vi "Agilent Tester.vi"() -> ()   [LabVIEW 2016]
uses:
  Type Definitions/WILT Agilent Data Cluster.ctl
  Type Definitions/WILT Agilent Channel Definition.ctl
panel:
  out "Agilent":T1
  in  "Open/Close (F:Close)":bool=TRUE
  in  "Open Valve":bool
  in  "Station":i32=1
  in  "Agilent Channels In":T2[](array[typedef])=[{"Channel"="301", "Station"="1", "Label"="Water Valve", "Agilent Station"="2", "Data"=0.0}, {"Channel"="302", "Station"="2", "Label"="Water Valve", "Agilent Station"="2", "Data"=0.0}, {"Channel"="303", "Station"="3", "Label"="Water Valve", "Agilent Station"="2", "Data"=0.0}, {"Channel"="304", "Station"="4", "Label"="Water Valve", "Agilent Station"="2", "Data"=0.0}, {"Channel"="305", "Station"="5", "Label"="Water Valve", "Agilent Station"="2", "Data"=0.0}, {"Channel"="306", "Station"="6", "Label"="Water Valve", "Agilent Station"="2", "Data"=0.0}, {"Channel"="307", "Station"="7", "Label"="Water Valve", "Agilent Station"="2", "Data"=0.0}, {"Channel"="308", "Station"="8", "Label"="Water Valve", "Agilent Station"="2", "Data"=0.0}, {"Channel"="309", "Station"="9", "Label"="Water Valve", "Agilent Station"="2", "Data"=0.0}, {"Channel"="310", "Station"="10", "Label"="Water Valve", "Agilent Station"="2", "Data"=0.0}, {"Channel"="311", "Station"="11", "Label"="Water Valve", "Agilent Station"="2", "Data"=0.0}, {"Channel"="312", "Station"="12", "Label"="Water Valve", "Agilent Station"="2", "Data"=0.0}, {"Channel"="313", "Station"="13", "Label"="Water Valve", "Agilent Station"="2", "Data"=0.0}, {"Channel"="314", "Station"="14", "Label"="Water Valve", "Agilent Station"="2", "Data"=0.0}, {"Channel"="315", "Station"="15", "Label"="Water Valve", "Agilent Station"="2", "Data"=0.0}, {"Channel"="316", "Station"="16", "Label"="Water Valve", "Agilent Station"="2", "Data"=0.0}, {"Channel"="317", "Station"="17", "Label"="Water Valve", "Agilent Station"="2", "Data"=0.0}, {"Channel"="318", "Station"="18", "Label"="Water Valve", "Agilent Station"="2", "Data"=0.0}, {"Channel"="319", "Station"="19", "Label"="Water Valve", "Agilent Station"="2", "Data"=0.0}, {"Channel"="320", "Station"="20", "Label"="Water Valve", "Agilent Station"="2", "Data"=0.0}, {"Channel"="101", "Station"="21", "Label"="Water Valve", "Agilent Station"="3", "Data"=0.0}, {"Channel"="102", "Station"="22", "Label"="Water Valve", "Agilent Station"="3", "Data"=0.0}, {"Channel"="103", "Station"="23", "Label"="Water Valve", "Agilent Station"="3", "Data"=0.0}, {"Channel"="104", "Station"="24", "Label"="Water Valve", "Agilent Station"="3", "Data"=0.0}, {"Channel"="105", "Station"="25", "Label"="Water Valve", "Agilent Station"="3", "Data"=0.0}, {"Channel"="106", "Station"="26", "Label"="Water Valve", "Agilent Station"="3", "Data"=0.0}, {"Channel"="107", "Station"="27", "Label"="Water Valve", "Agilent Station"="3", "Data"=0.0}, {"Channel"="108", "Station"="28", "Label"="Water Valve", "Agilent Station"="3", "Data"=0.0}, {"Channel"="109", "Station"="29", "Label"="Water Valve", "Agilent Station"="3", "Data"=0.0}, {"Channel"="110", "Station"="30", "Label"="Water Valve", "Agilent Station"="3", "Data"=0.0}, {"Channel"="111", "Station"="31", "Label"="Water Valve", "Agilent Station"="3", "Data"=0.0}, {"Channel"="112", "Station"="32", "Label"="Water Valve", "Agilent Station"="3", "Data"=0.0}, {"Channel"="101", "Station"="33", "Label"="Water Valve", "Agilent Station"="5", "Data"=0.0}, {"Channel"="102", "Station"="34", "Label"="Water Valve", "Agilent Station"="5", "Data"=0.0}, {"Channel"="103", "Station"="35", "Label"="Water Valve", "Agilent Station"="5", "Data"=0.0}, {"Channel"="104", "Station"="36", "Label"="Water Valve", "Agilent Station"="5", "Data"=0.0}, {"Channel"="105", "Station"="37", "Label"="Water Valve", "Agilent Station"="5", "Data"=0.0}, {"Channel"="106", "Station"="38", "Label"="Water Valve", "Agilent Station"="5", "Data"=0.0}, {"Channel"="107", "Station"="39", "Label"="Water Valve", "Agilent Station"="5", "Data"=0.0}, {"Channel"="108", "Station"="40", "Label"="Water Valve", "Agilent Station"="5", "Data"=0.0}, {"Channel"="109", "Station"="41", "Label"="Water Valve", "Agilent Station"="5", "Data"=0.0}, {"Channel"="110", "Station"="42", "Label"="Water Valve", "Agilent Station"="5", "Data"=0.0}, {"Channel"="111", "Station"="43", "Label"="Water Valve", "Agilent Station"="5", "Data"=0.0}, {"Channel"="112", "Station"="44", "Label"="Water Valve", "Agilent Station"="5", "Data"=0.0}, {"Channel"="113", "Station"="45", "Label"="Water Valve", "Agilent Station"="5", "Data"=0.0}, {"Channel"="114", "Station"="46", "Label"="Water Valve", "Agilent Station"="5", "Data"=0.0}, {"Channel"="115", "Station"="47", "Label"="Water Valve", "Agilent Station"="5", "Data"=0.0}, {"Channel"="116", "Station"="48", "Label"="Water Valve", "Agilent Station"="5", "Data"=0.0}, {"Channel"="117", "Station"="49", "Label"="Water Valve", "Agilent Station"="5", "Data"=0.0}, {"Channel"="118", "Station"="50", "Label"="Water Valve", "Agilent Station"="5", "Data"=0.0}, {"Channel"="119", "Station"="51", "Label"="Water Valve", "Agilent Station"="5", "Data"=0.0}, {"Channel"="120", "Station"="52", "Label"="Water Valve", "Agilent Station"="5", "Data"=0.0}, {"Channel"="201", "Station"="53", "Label"="Water Valve", "Agilent Station"="5", "Data"=0.0}, {"Channel"="202", "Station"="54", "Label"="Water Valve", "Agilent Station"="5", "Data"=0.0}, {"Channel"="203", "Station"="55", "Label"="Water Valve", "Agilent Station"="5", "Data"=0.0}, {"Channel"="204", "Station"="56", "Label"="Water Valve", "Agilent Station"="5", "Data"=0.0}, {"Channel"="301", "Station"="21", "Label"="Start Button", "Agilent Station"="5", "Data"=0.0}, {"Channel"="302", "Station"="22", "Label"="Start Button", "Agilent Station"="5", "Data"=0.0}, {"Channel"="303", "Station"="23", "Label"="Start Button", "Agilent Station"="5", "Data"=0.0}, {"Channel"="304", "Station"="24", "Label"="Start Button", "Agilent Station"="5", "Data"=0.0}, {"Channel"="305", "Station"="25", "Label"="Start Button", "Agilent Station"="5", "Data"=0.0}, {"Channel"="306", "Station"="26", "Label"="Start Button", "Agilent Station"="5", "Data"=0.0}, {"Channel"="307", "Station"="27", "Label"="Start Button", "Agilent Station"="5", "Data"=0.0}, {"Channel"="308", "Station"="28", "Label"="Start Button", "Agilent Station"="5", "Data"=0.0}, {"Channel"="309", "Station"="29", "Label"="Start Button", "Agilent Station"="5", "Data"=0.0}, {"Channel"="310", "Station"="30", "Label"="Start Button", "Agilent Station"="5", "Data"=0.0}, {"Channel"="311", "Station"="31", "Label"="Start Button", "Agilent Station"="5", "Data"=0.0}, {"Channel"="312", "Station"="32", "Label"="Start Button", "Agilent Station"="5", "Data"=0.0}, {"Channel"="101", "Station"="33", "Label"="Start Button", "Agilent Station"="7", "Data"=0.0}, {"Channel"="102", "Station"="34", "Label"="Start Button", "Agilent Station"="7", "Data"=0.0}, {"Channel"="103", "Station"="35", "Label"="Start Button", "Agilent Station"="7", "Data"=0.0}, {"Channel"="104", "Station"="36", "Label"="Start Button", "Agilent Station"="7", "Data"=0.0}, {"Channel"="105", "Station"="37", "Label"="Start Button", "Agilent Station"="7", "Data"=0.0}, {"Channel"="106", "Station"="38", "Label"="Start Button", "Agilent Station"="7", "Data"=0.0}, {"Channel"="107", "Station"="39", "Label"="Start Button", "Agilent Station"="7", "Data"=0.0}, {"Channel"="108", "Station"="40", "Label"="Start Button", "Agilent Station"="7", "Data"=0.0}, {"Channel"="109", "Station"="41", "Label"="Start Button", "Agilent Station"="7", "Data"=0.0}, {"Channel"="110", "Station"="42", "Label"="Start Button", "Agilent Station"="7", "Data"=0.0}, {"Channel"="111", "Station"="43", "Label"="Start Button", "Agilent Station"="7", "Data"=0.0}, {"Channel"="112", "Station"="44", "Label"="Start Button", "Agilent Station"="7", "Data"=0.0}]
  in  "Data Out Array":T3=[{"Channel"="101", "Station"="1", "Label"="L1 Current", "Agilent Station"="1", "Data"=0.0}, {"Channel"="102", "Station"="1", "Label"="L2 Current", "Agilent Station"="1", "Data"=0.0}, {"Channel"="103", "Station"="2", "Label"="L1 Current", "Agilent Station"="1", "Data"=0.0}, {"Channel"="104", "Station"="2", "Label"="L2 Current", "Agilent Station"="1", "Data"=0.0}, {"Channel"="105", "Station"="3", "Label"="L1 Current", "Agilent Station"="1", "Data"=0.0}, {"Channel"="106", "Station"="3", "Label"="L2 Current", "Agilent Station"="1", "Data"=0.0}, {"Channel"="107", "Station"="4", "Label"="L1 Current", "Agilent Station"="1", "Data"=0.0}, {"Channel"="108", "Station"="4", "Label"="L2 Current", "Agilent Station"="1", "Data"=0.0}, {"Channel"="109", "Station"="5", "Label"="L1 Current", "Agilent Station"="1", "Data"=0.0}, {"Channel"="110", "Station"="5", "Label"="L2 Current", "Agilent Station"="1", "Data"=0.0}, {"Channel"="111", "Station"="6", "Label"="L1 Current", "Agilent Station"="1", "Data"=0.0}, {"Channel"="112", "Station"="6", "Label"="L2 Current", "Agilent Station"="1", "Data"=0.0}, {"Channel"="113", "Station"="7", "Label"="L1 Current", "Agilent Station"="1", "Data"=0.0}, {"Channel"="114", "Station"="7", "Label"="L2 Current", "Agilent Station"="1", "Data"=0.0}, {"Channel"="115", "Station"="8", "Label"="L1 Current", "Agilent Station"="1", "Data"=0.0}, {"Channel"="116", "Station"="8", "Label"="L2 Current", "Agilent Station"="1", "Data"=0.0}, {"Channel"="201", "Station"="9", "Label"="L1 Current", "Agilent Station"="1", "Data"=0.0}, {"Channel"="202", "Station"="9", "Label"="L2 Current", "Agilent Station"="1", "Data"=0.0}, {"Channel"="203", "Station"="10", "Label"="L1 Current", "Agilent Station"="1", "Data"=0.0}, {"Channel"="204", "Station"="10", "Label"="L2 Current", "Agilent Station"="1", "Data"=0.0}, {"Channel"="205", "Station"="11", "Label"="L1 Current", "Agilent Station"="1", "Data"=0.0}, {"Channel"="206", "Station"="11", "Label"="L2 Current", "Agilent Station"="1", "Data"=0.0}, {"Channel"="207", "Station"="12", "Label"="L1 Current", "Agilent Station"="1", "Data"=0.0}, {"Channel"="208", "Station"="12", "Label"="L2 Current", "Agilent Station"="1", "Data"=0.0}, {"Channel"="209", "Station"="13", "Label"="L1 Current", "Agilent Station"="1", "Data"=0.0}, {"Channel"="210", "Station"="13", "Label"="L2 Current", "Agilent Station"="1", "Data"=0.0}, {"Channel"="211", "Station"="14", "Label"="L1 Current", "Agilent Station"="1", "Data"=0.0}, {"Channel"="212", "Station"="14", "Label"="L2 Current", "Agilent Station"="1", "Data"=0.0}, {"Channel"="213", "Station"="15", "Label"="L1 Current", "Agilent Station"="1", "Data"=0.0}, {"Channel"="214", "Station"="15", "Label"="L2 Current", "Agilent Station"="1", "Data"=0.0}, {"Channel"="215", "Station"="16", "Label"="L1 Current", "Agilent Station"="1", "Data"=0.0}, {"Channel"="216", "Station"="16", "Label"="L2 Current", "Agilent Station"="1", "Data"=0.0}, {"Channel"="301", "Station"="17", "Label"="L1 Current", "Agilent Station"="1", "Data"=0.0}, {"Channel"="302", "Station"="17", "Label"="L2 Current", "Agilent Station"="1", "Data"=0.0}, {"Channel"="303", "Station"="18", "Label"="L1 Current", "Agilent Station"="1", "Data"=0.0}, {"Channel"="304", "Station"="18", "Label"="L2 Current", "Agilent Station"="1", "Data"=0.0}, {"Channel"="305", "Station"="19", "Label"="L1 Current", "Agilent Station"="1", "Data"=0.0}, {"Channel"="306", "Station"="19", "Label"="L2 Current", "Agilent Station"="1", "Data"=0.0}, {"Channel"="307", "Station"="20", "Label"="L1 Current", "Agilent Station"="1", "Data"=0.0}, {"Channel"="308", "Station"="20", "Label"="L2 Current", "Agilent Station"="1", "Data"=0.0}, {"Channel"="309", "Station"="21", "Label"="L1 Current", "Agilent Station"="1", "Data"=0.0}, {"Channel"="310", "Station"="21", "Label"="L2 Current", "Agilent Station"="1", "Data"=0.0}, {"Channel"="311", "Station"="22", "Label"="L1 Current", "Agilent Station"="1", "Data"=0.0}, {"Channel"="312", "Station"="22", "Label"="L2 Current", "Agilent Station"="1", "Data"=0.0}, {"Channel"="313", "Station"="23", "Label"="L1 Current", "Agilent Station"="1", "Data"=0.0}, {"Channel"="314", "Station"="23", "Label"="L2 Current", "Agilent Station"="1", "Data"=0.0}, {"Channel"="315", "Station"="24", "Label"="L1 Current", "Agilent Station"="1", "Data"=0.0}, {"Channel"="316", "Station"="24", "Label"="L2 Current", "Agilent Station"="1", "Data"=0.0}, {"Channel"="101", "Station"="25", "Label"="L1 Current", "Agilent Station"="2", "Data"=0.0}, {"Channel"="102", "Station"="25", "Label"="L2 Current", "Agilent Station"="2", "Data"=0.0}, {"Channel"="103", "Station"="26", "Label"="L1 Current", "Agilent Station"="2", "Data"=0.0}, {"Channel"="104", "Station"="26", "Label"="L2 Current", "Agilent Station"="2", "Data"=0.0}, {"Channel"="105", "Station"="27", "Label"="L1 Current", "Agilent Station"="2", "Data"=0.0}, {"Channel"="106", "Station"="27", "Label"="L2 Current", "Agilent Station"="2", "Data"=0.0}, {"Channel"="107", "Station"="28", "Label"="L1 Current", "Agilent Station"="2", "Data"=0.0}, {"Channel"="108", "Station"="28", "Label"="L2 Current", "Agilent Station"="2", "Data"=0.0}, {"Channel"="109", "Station"="29", "Label"="L1 Current", "Agilent Station"="2", "Data"=0.0}, {"Channel"="110", "Station"="29", "Label"="L2 Current", "Agilent Station"="2", "Data"=0.0}, {"Channel"="111", "Station"="30", "Label"="L1 Current", "Agilent Station"="2", "Data"=0.0}, {"Channel"="112", "Station"="30", "Label"="L2 Current", "Agilent Station"="2", "Data"=0.0}, {"Channel"="113", "Station"="31", "Label"="L1 Current", "Agilent Station"="2", "Data"=0.0}, {"Channel"="114", "Station"="31", "Label"="L2 Current", "Agilent Station"="2", "Data"=0.0}, {"Channel"="115", "Station"="32", "Label"="L1 Current", "Agilent Station"="2", "Data"=0.0}, {"Channel"="116", "Station"="32", "Label"="L2 Current", "Agilent Station"="2", "Data"=0.0}, {"Channel"="201", "Station"="5", "Label"="Volts", "Agilent Station"="2", "Data"=0.0}, {"Channel"="202", "Station"="6", "Label"="Volts", "Agilent Station"="2", "Data"=0.0}, {"Channel"="203", "Station"="7", "Label"="Volts", "Agilent Station"="2", "Data"=0.0}, {"Channel"="204", "Station"="8", "Label"="Volts", "Agilent Station"="2", "Data"=0.0}, {"Channel"="205", "Station"="9", "Label"="Volts", "Agilent Station"="2", "Data"=0.0}, {"Channel"="206", "Station"="10", "Label"="Volts", "Agilent Station"="2", "Data"=0.0}, {"Channel"="207", "Station"="11", "Label"="Volts", "Agilent Station"="2", "Data"=0.0}, {"Channel"="208", "Station"="12", "Label"="Volts", "Agilent Station"="2", "Data"=0.0}, {"Channel"="209", "Station"="13", "Label"="Volts", "Agilent Station"="2", "Data"=0.0}, {"Channel"="210", "Station"="14", "Label"="Volts", "Agilent Station"="2", "Data"=0.0}, {"Channel"="211", "Station"="21", "Label"="Volts", "Agilent Station"="2", "Data"=0.0}, {"Channel"="211", "Station"="22", "Label"="Volts", "Agilent Station"="2", "Data"=0.0}, {"Channel"="211", "Station"="23", "Label"="Volts", "Agilent Station"="2", "Data"=0.0}, {"Channel"="212", "Station"="24", "Label"="Volts", "Agilent Station"="2", "Data"=0.0}, {"Channel"="212", "Station"="25", "Label"="Volts", "Agilent Station"="2", "Data"=0.0}, {"Channel"="212", "Station"="26", "Label"="Volts", "Agilent Station"="2", "Data"=0.0}, {"Channel"="213", "Station"="27", "Label"="Volts", "Agilent Station"="2", "Data"=0.0}, {"Channel"="213", "Station"="28", "Label"="Volts", "Agilent Station"="2", "Data"=0.0}, {"Channel"="213", "Station"="29", "Label"="Volts", "Agilent Station"="2", "Data"=0.0}, {"Channel"="214", "Station"="30", "Label"="Volts", "Agilent Station"="2", "Data"=0.0}, {"Channel"="214", "Station"="31", "Label"="Volts", "Agilent Station"="2", "Data"=0.0}, {"Channel"="214", "Station"="32", "Label"="Volts", "Agilent Station"="2", "Data"=0.0}, {"Channel"="215", "Station"="15", "Label"="Volts", "Agilent Station"="2", "Data"=0.0}, {"Channel"="216", "Station"="16", "Label"="Volts", "Agilent Station"="2", "Data"=0.0}, {"Channel"="201", "Station"="1", "Label"="Temperature", "Agilent Station"="3", "Data"=0.0}, {"Channel"="202", "Station"="2", "Label"="Temperature", "Agilent Station"="3", "Data"=0.0}, {"Channel"="203", "Station"="3", "Label"="Temperature", "Agilent Station"="3", "Data"=0.0}, {"Channel"="204", "Station"="4", "Label"="Temperature", "Agilent Station"="3", "Data"=0.0}, {"Channel"="205", "Station"="5", "Label"="Temperature", "Agilent Station"="3", "Data"=0.0}, {"Channel"="206", "Station"="6", "Label"="Temperature", "Agilent Station"="3", "Data"=0.0}, {"Channel"="207", "Station"="7", "Label"="Temperature", "Agilent Station"="3", "Data"=0.0}, {"Channel"="208", "Station"="8", "Label"="Temperature", "Agilent Station"="3", "Data"=0.0}, {"Channel"="209", "Station"="9", "Label"="Temperature", "Agilent Station"="3", "Data"=0.0}, {"Channel"="210", "Station"="10", "Label"="Temperature", "Agilent Station"="3", "Data"=0.0}, {"Channel"="211", "Station"="11", "Label"="Temperature", "Agilent Station"="3", "Data"=0.0}, {"Channel"="212", "Station"="12", "Label"="Temperature", "Agilent Station"="3", "Data"=0.0}, {"Channel"="213", "Station"="13", "Label"="Temperature", "Agilent Station"="3", "Data"=0.0}, {"Channel"="214", "Station"="14", "Label"="Temperature", "Agilent Station"="3", "Data"=0.0}, {"Channel"="215", "Station"="15", "Label"="Temperature", "Agilent Station"="3", "Data"=0.0}, {"Channel"="216", "Station"="16", "Label"="Temperature", "Agilent Station"="3", "Data"=0.0}, {"Channel"="217", "Station"="17", "Label"="Temperature", "Agilent Station"="3", "Data"=0.0}, {"Channel"="218", "Station"="18", "Label"="Temperature", "Agilent Station"="3", "Data"=0.0}, {"Channel"="219", "Station"="19", "Label"="Temperature", "Agilent Station"="3", "Data"=0.0}, {"Channel"="220", "Station"="20", "Label"="Temperature", "Agilent Station"="3", "Data"=0.0}, {"Channel"="301", "Station"="21", "Label"="Temperature", "Agilent Station"="3", "Data"=0.0}, {"Channel"="302", "Station"="22", "Label"="Temperature", "Agilent Station"="3", "Data"=0.0}, {"Channel"="303", "Station"="23", "Label"="Temperature", "Agilent Station"="3", "Data"=0.0}, {"Channel"="304", "Station"="24", "Label"="Temperature", "Agilent Station"="3", "Data"=0.0}, {"Channel"="305", "Station"="25", "Label"="Temperature", "Agilent Station"="3", "Data"=0.0}, {"Channel"="306", "Station"="26", "Label"="Temperature", "Agilent Station"="3", "Data"=0.0}, {"Channel"="307", "Station"="27", "Label"="Temperature", "Agilent Station"="3", "Data"=0.0}, {"Channel"="308", "Station"="28", "Label"="Temperature", "Agilent Station"="3", "Data"=0.0}, {"Channel"="309", "Station"="29", "Label"="Temperature", "Agilent Station"="3", "Data"=0.0}, {"Channel"="310", "Station"="30", "Label"="Temperature", "Agilent Station"="3", "Data"=0.0}, {"Channel"="311", "Station"="31", "Label"="Temperature", "Agilent Station"="3", "Data"=0.0}, {"Channel"="312", "Station"="32", "Label"="Temperature", "Agilent Station"="3", "Data"=0.0}, {"Channel"="313", "Station"="1", "Label"="Volts", "Agilent Station"="3", "Data"=0.0}, {"Channel"="314", "Station"="2", "Label"="Volts", "Agilent Station"="3", "Data"=0.0}, {"Channel"="315", "Station"="3", "Label"="Volts", "Agilent Station"="3", "Data"=0.0}, {"Channel"="316", "Station"="4", "Label"="Volts", "Agilent Station"="3", "Data"=0.0}, {"Channel"="101", "Station"="33", "Label"="L1 Current", "Agilent Station"="4", "Data"=0.0}, {"Channel"="102", "Station"="33", "Label"="L2 Current", "Agilent Station"="4", "Data"=0.0}, {"Channel"="103", "Station"="34", "Label"="L1 Current", "Agilent Station"="4", "Data"=0.0}, {"Channel"="104", "Station"="34", "Label"="L2 Current", "Agilent Station"="4", "Data"=0.0}, {"Channel"="105", "Station"="35", "Label"="L1 Current", "Agilent Station"="4", "Data"=0.0}, {"Channel"="106", "Station"="35", "Label"="L2 Current", "Agilent Station"="4", "Data"=0.0}, {"Channel"="107", "Station"="36", "Label"="L1 Current", "Agilent Station"="4", "Data"=0.0}, {"Channel"="108", "Station"="36", "Label"="L2 Current", "Agilent Station"="4", "Data"=0.0}, {"Channel"="109", "Station"="37", "Label"="L1 Current", "Agilent Station"="4", "Data"=0.0}, {"Channel"="110", "Station"="37", "Label"="L2 Current", "Agilent Station"="4", "Data"=0.0}, {"Channel"="111", "Station"="38", "Label"="L1 Current", "Agilent Station"="4", "Data"=0.0}, {"Channel"="112", "Station"="38", "Label"="L2 Current", "Agilent Station"="4", "Data"=0.0}, {"Channel"="113", "Station"="39", "Label"="L1 Current", "Agilent Station"="4", "Data"=0.0}, {"Channel"="114", "Station"="39", "Label"="L2 Current", "Agilent Station"="4", "Data"=0.0}, {"Channel"="115", "Station"="40", "Label"="L1 Current", "Agilent Station"="4", "Data"=0.0}, {"Channel"="116", "Station"="40", "Label"="L2 Current", "Agilent Station"="4", "Data"=0.0}, {"Channel"="201", "Station"="41", "Label"="L1 Current", "Agilent Station"="4", "Data"=0.0}, {"Channel"="202", "Station"="41", "Label"="L2 Current", "Agilent Station"="4", "Data"=0.0}, {"Channel"="203", "Station"="42", "Label"="L1 Current", "Agilent Station"="4", "Data"=0.0}, {"Channel"="204", "Station"="42", "Label"="L2 Current", "Agilent Station"="4", "Data"=0.0}, {"Channel"="205", "Station"="43", "Label"="L1 Current", "Agilent Station"="4", "Data"=0.0}, {"Channel"="206", "Station"="43", "Label"="L2 Current", "Agilent Station"="4", "Data"=0.0}, {"Channel"="207", "Station"="44", "Label"="L1 Current", "Agilent Station"="4", "Data"=0.0}, {"Channel"="208", "Station"="44", "Label"="L2 Current", "Agilent Station"="4", "Data"=0.0}, {"Channel"="209", "Station"="45", "Label"="L1 Current", "Agilent Station"="4", "Data"=0.0}, {"Channel"="210", "Station"="45", "Label"="L2 Current", "Agilent Station"="4", "Data"=0.0}, {"Channel"="211", "Station"="46", "Label"="L1 Current", "Agilent Station"="4", "Data"=0.0}, {"Channel"="212", "Station"="46", "Label"="L2 Current", "Agilent Station"="4", "Data"=0.0}, {"Channel"="213", "Station"="47", "Label"="L1 Current", "Agilent Station"="4", "Data"=0.0}, {"Channel"="214", "Station"="47", "Label"="L2 Current", "Agilent Station"="4", "Data"=0.0}, {"Channel"="215", "Station"="48", "Label"="L1 Current", "Agilent Station"="4", "Data"=0.0}, {"Channel"="216", "Station"="48", "Label"="L2 Current", "Agilent Station"="4", "Data"=0.0}, {"Channel"="301", "Station"="49", "Label"="L1 Current", "Agilent Station"="4", "Data"=0.0}, {"Channel"="302", "Station"="49", "Label"="L2 Current", "Agilent Station"="4", "Data"=0.0}, {"Channel"="303", "Station"="50", "Label"="L1 Current", "Agilent Station"="4", "Data"=0.0}, {"Channel"="304", "Station"="50", "Label"="L2 Current", "Agilent Station"="4", "Data"=0.0}, {"Channel"="305", "Station"="51", "Label"="L1 Current", "Agilent Station"="4", "Data"=0.0}, {"Channel"="306", "Station"="51", "Label"="L2 Current", "Agilent Station"="4", "Data"=0.0}, {"Channel"="307", "Station"="52", "Label"="L1 Current", "Agilent Station"="4", "Data"=0.0}, {"Channel"="308", "Station"="52", "Label"="L2 Current", "Agilent Station"="4", "Data"=0.0}, {"Channel"="309", "Station"="53", "Label"="L1 Current", "Agilent Station"="4", "Data"=0.0}, {"Channel"="310", "Station"="53", "Label"="L2 Current", "Agilent Station"="4", "Data"=0.0}, {"Channel"="311", "Station"="54", "Label"="L1 Current", "Agilent Station"="4", "Data"=0.0}, {"Channel"="312", "Station"="54", "Label"="L2 Current", "Agilent Station"="4", "Data"=0.0}, {"Channel"="313", "Station"="55", "Label"="L1 Current", "Agilent Station"="4", "Data"=0.0}, {"Channel"="314", "Station"="55", "Label"="L2 Current", "Agilent Station"="4", "Data"=0.0}, {"Channel"="315", "Station"="56", "Label"="L1 Current", "Agilent Station"="4", "Data"=0.0}, {"Channel"="316", "Station"="56", "Label"="L2 Current", "Agilent Station"="4", "Data"=0.0}, {"Channel"="101", "Station"="33", "Label"="Temperature", "Agilent Station"="6", "Data"=0.0}, {"Channel"="102", "Station"="34", "Label"="Temperature", "Agilent Station"="6", "Data"=0.0}, {"Channel"="103", "Station"="35", "Label"="Temperature", "Agilent Station"="6", "Data"=0.0}, {"Channel"="104", "Station"="36", "Label"="Temperature", "Agilent Station"="6", "Data"=0.0}, {"Channel"="105", "Station"="37", "Label"="Temperature", "Agilent Station"="6", "Data"=0.0}, {"Channel"="106", "Station"="38", "Label"="Temperature", "Agilent Station"="6", "Data"=0.0}, {"Channel"="107", "Station"="39", "Label"="Temperature", "Agilent Station"="6", "Data"=0.0}, {"Channel"="108", "Station"="40", "Label"="Temperature", "Agilent Station"="6", "Data"=0.0}, {"Channel"="109", "Station"="41", "Label"="Temperature", "Agilent Station"="6", "Data"=0.0}, {"Channel"="110", "Station"="42", "Label"="Temperature", "Agilent Station"="6", "Data"=0.0}, {"Channel"="111", "Station"="43", "Label"="Temperature", "Agilent Station"="6", "Data"=0.0}, {"Channel"="112", "Station"="44", "Label"="Temperature", "Agilent Station"="6", "Data"=0.0}, {"Channel"="113", "Station"="45", "Label"="Temperature", "Agilent Station"="6", "Data"=0.0}, {"Channel"="114", "Station"="46", "Label"="Temperature", "Agilent Station"="6", "Data"=0.0}, {"Channel"="115", "Station"="47", "Label"="Temperature", "Agilent Station"="6", "Data"=0.0}, {"Channel"="116", "Station"="48", "Label"="Temperature", "Agilent Station"="6", "Data"=0.0}, {"Channel"="117", "Station"="49", "Label"="Temperature", "Agilent Station"="6", "Data"=0.0}, {"Channel"="118", "Station"="50", "Label"="Temperature", "Agilent Station"="6", "Data"=0.0}, {"Channel"="119", "Station"="51", "Label"="Temperature", "Agilent Station"="6", "Data"=0.0}, {"Channel"="120", "Station"="52", "Label"="Temperature", "Agilent Station"="6", "Data"=0.0}, {"Channel"="201", "Station"="53", "Label"="Temperature", "Agilent Station"="6", "Data"=0.0}, {"Channel"="202", "Station"="54", "Label"="Temperature", "Agilent Station"="6", "Data"=0.0}, {"Channel"="203", "Station"="55", "Label"="Temperature", "Agilent Station"="6", "Data"=0.0}, {"Channel"="204", "Station"="56", "Label"="Temperature", "Agilent Station"="6", "Data"=0.0}, {"Channel"="205", "Station"="33", "Label"="Volts", "Agilent Station"="6", "Data"=0.0}, {"Channel"="205", "Station"="34", "Label"="Volts", "Agilent Station"="6", "Data"=0.0}, {"Channel"="205", "Station"="35", "Label"="Volts", "Agilent Station"="6", "Data"=0.0}, {"Channel"="206", "Station"="36", "Label"="Volts", "Agilent Station"="6", "Data"=0.0}, {"Channel"="206", "Station"="37", "Label"="Volts", "Agilent Station"="6", "Data"=0.0}, {"Channel"="206", "Station"="38", "Label"="Volts", "Agilent Station"="6", "Data"=0.0}, {"Channel"="207", "Station"="39", "Label"="Volts", "Agilent Station"="6", "Data"=0.0}, {"Channel"="207", "Station"="40", "Label"="Volts", "Agilent Station"="6", "Data"=0.0}, {"Channel"="208", "Station"="42", "Label"="Volts", "Agilent Station"="6", "Data"=0.0}, {"Channel"="208", "Station"="43", "Label"="Volts", "Agilent Station"="6", "Data"=0.0}, {"Channel"="208", "Station"="44", "Label"="Volts", "Agilent Station"="6", "Data"=0.0}, {"Channel"="209", "Station"="45", "Label"="Volts", "Agilent Station"="6", "Data"=0.0}, {"Channel"="209", "Station"="46", "Label"="Volts", "Agilent Station"="6", "Data"=0.0}, {"Channel"="209", "Station"="47", "Label"="Volts", "Agilent Station"="6", "Data"=0.0}, {"Channel"="210", "Station"="45", "Label"="Volts (208)", "Agilent Station"="6", "Data"=0.0}, {"Channel"="211", "Station"="45", "Label"="SW (208)", "Agilent Station"="6", "Data"=0.0}, {"Channel"="212", "Station"="48", "Label"="Volts", "Agilent Station"="6", "Data"=0.0}, {"Channel"="212", "Station"="49", "Label"="Volts", "Agilent Station"="6", "Data"=0.0}, {"Channel"="212", "Station"="50", "Label"="Volts", "Agilent Station"="6", "Data"=0.0}, {"Channel"="213", "Station"="48", "Label"="SW (208)", "Agilent Station"="6", "Data"=0.0}, {"Channel"="214", "Station"="51", "Label"="Volts (208)", "Agilent Station"="6", "Data"=0.0}, {"Channel"="215", "Station"="51", "Label"="SW (208)", "Agilent Station"="6", "Data"=0.0}, {"Channel"="216", "Station"="54", "Label"="Volts", "Agilent Station"="6", "Data"=0.0}, {"Channel"="216", "Station"="55", "Label"="Volts", "Agilent Station"="6", "Data"=0.0}, {"Channel"="216", "Station"="56", "Label"="Volts", "Agilent Station"="6", "Data"=0.0}, {"Channel"="301", "Station"="17", "Label"="Volts", "Agilent Station"="6", "Data"=0.0}, {"Channel"="302", "Station"="18", "Label"="Volts", "Agilent Station"="6", "Data"=0.0}, {"Channel"="303", "Station"="19", "Label"="Volts", "Agilent Station"="6", "Data"=0.0}, {"Channel"="304", "Station"="20", "Label"="Volts", "Agilent Station"="6", "Data"=0.0}, {"Channel"="305", "Station"="51", "Label"="Volts", "Agilent Station"="6", "Data"=0.0}, {"Channel"="305", "Station"="52", "Label"="Volts", "Agilent Station"="6", "Data"=0.0}, {"Channel"="305", "Station"="53", "Label"="Volts", "Agilent Station"="6", "Data"=0.0}, {"Channel"="306", "Station"="48", "Label"="Volts (208)", "Agilent Station"="6", "Data"=0.0}]
  out "Loop Time":u32=9107494
  out "Numeric":i32
  in  "stop":bool
  out "Output Data (Numbers Only)":dbl[](array[numeric])=[0.003303, 0.0082578, -0.003303, -0.003303, 0.0115608, 0.0115608, -0.0016515, 0.0148638, 0.0082578, 0.0066063, -0.0379854, -0.0016515, -0.0066063, -0.0016515, -0.003303, 0.0, -0.247731, 238.69858, 258.4842, 240.01984, 0.842289, 134.18836, 1.337751, 167.79744, 131.31466, 132.10741, 234.28894, 233.94212, 233.23195, 234.70183, -264.09781, -5.549199]
  in  "VISA Resource Name":refnum<visa-resource-name>="AGILENT2"
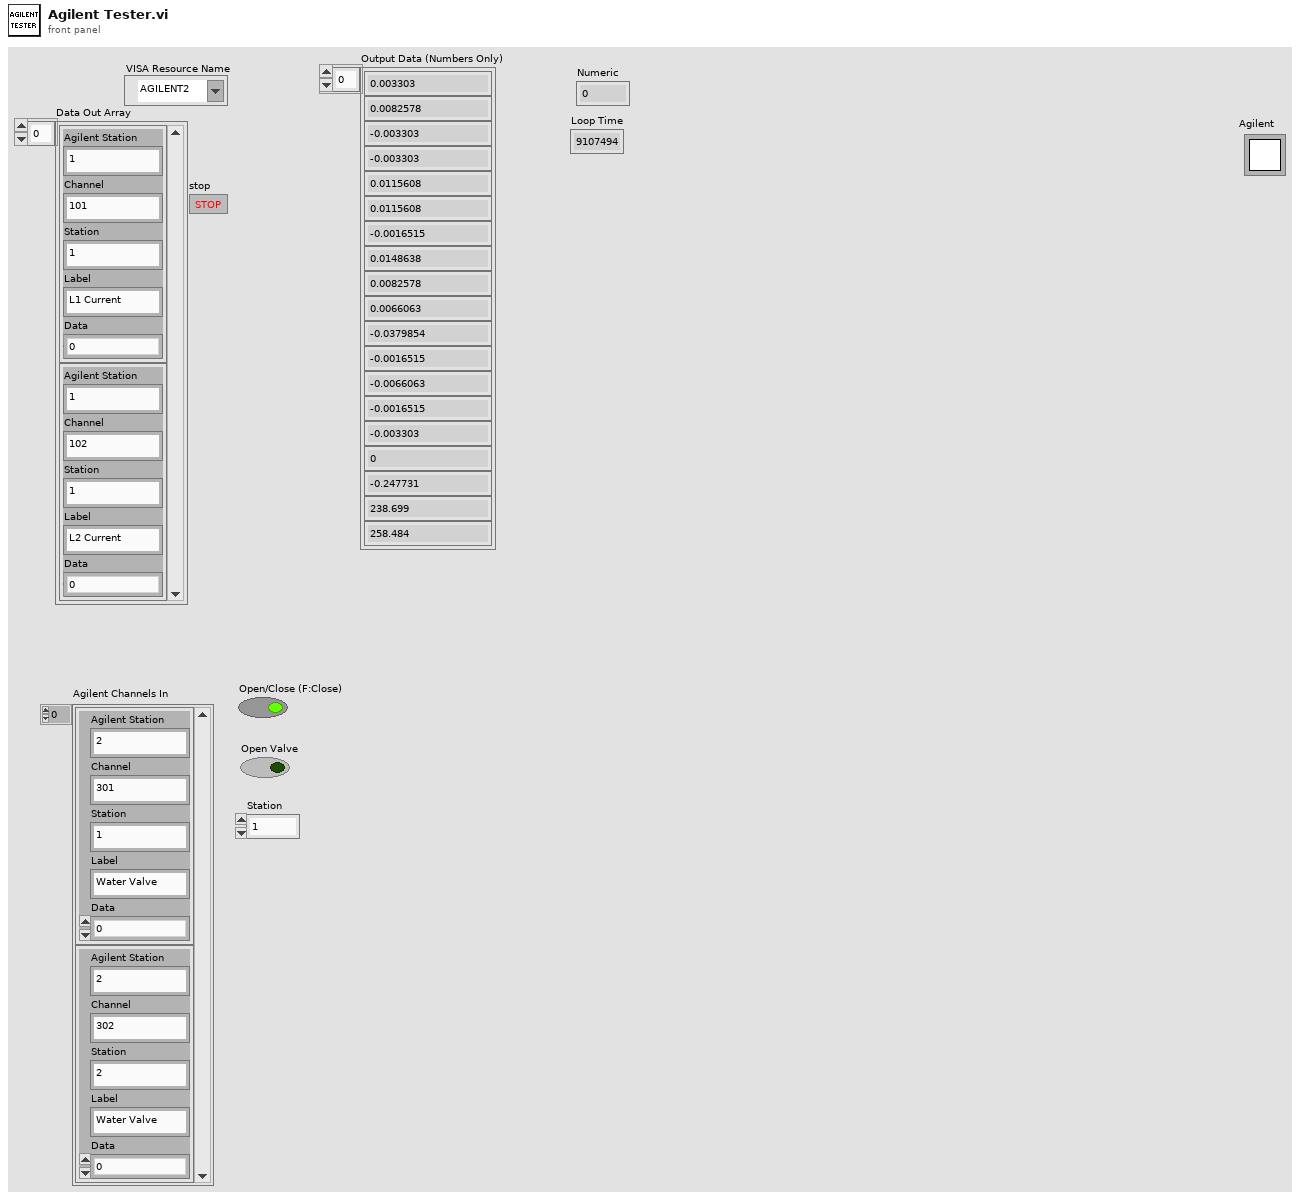
[diagram p1: front panel]
types:
  T1 = typedef "Semaphore RefNum" = refnum<k1>
  T2 = typedef "WILT Agilent Channel Definition.ctl" = cluster{"Channel":string, "Station":string, "Label":string, "Agilent Station":string, "Data":dbl}
  T3 = typedef "WILT Agilent Data Cluster.ctl" = T2[]
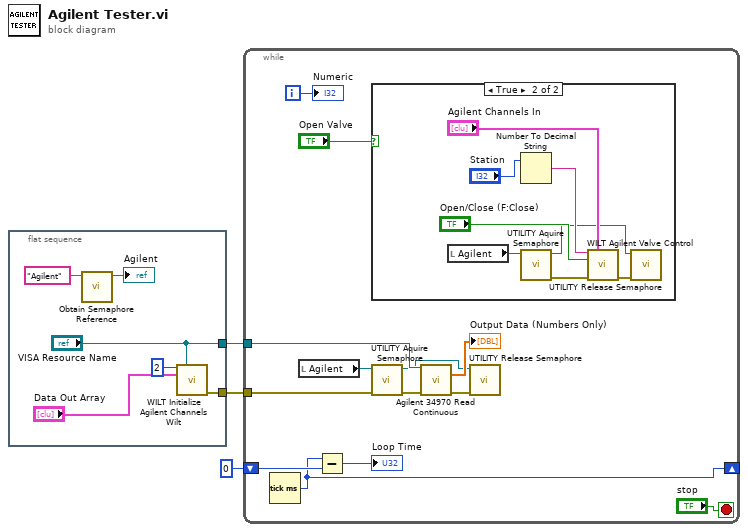
[diagram p0: block diagram]
diagram:
  n1 = flat-sequence {
    tunnel: ["VISA Resource Name"] -> w2
    tunnel: [w6] -> w1
    frame #0 {
      n2 = call <vilib>:"Obtain Semaphore Reference.vi"("name (unnamed)"="Agilent") -> ("semaphore"=→"Agilent":T1)  [unwired: 4 in, 2 out]
      n3 = call "WILT Initialize Agilent Channels Wilt.vi"("Agilent Number"=2, "VISA Resource Name"="VISA Resource Name", "Data Array"="Data Out Array") -> ("error out"=w6:errorcluster)  [unwired: 11 in, 1 out]
    }
  }
  n4 = while {
    tunnel: w2 -> [w22]
    shift-right: [w16] -> _
    shift-left: 0 -> [w18]
    tunnel: w1 -> [w13]
    i -> [w19]
    stop <- "stop" stop-if-true
    n5 = Tick Count (ms)() -> (millisecond timer value=w16:u32)
    n6 = local read "Agilent"() -> (w10:T1)
    n7 = Subtract(x=w16, y=w18) -> (x-y=→"Loop Time":u32)
    n8 = case shown="True" "Open Valve" {
      frame False {
      }
      frame True {
        n9 = local read "Agilent"() -> (w23:T1)
        n10 = Number To Decimal String(number="Station") -> (decimal integer string=w30:string)  [unwired: 1 in]
        n11 = call "UTILITY Aquire Semaphore.vi"("Refnum in"=w23) -> ("error out"=w26:errorcluster, "Refnum out"=w24:T1)  [unwired: 8 in, 1 out]
        n12 = call "WILT Agilent Valve Control.vi"("Station In"=w30, "Agilent Channels In"="Agilent Channels In", "Open/Close (F:Close)"="Open/Close (F:Close)", "error in (no error)"=w26) -> ("error out"=w25:errorcluster)  [unwired: 9 in, 2 out]
        n13 = call "UTILITY Release Semaphore.vi"("error in (no error)"=w25, "Refnum in"=w24) -> ()  [unwired: 9 in, 1 out]
      }
    }
    n14 = call "UTILITY Aquire Semaphore.vi"("error in (no error)"=w13, "Refnum in"=w10) -> ("error out"=w14:errorcluster, "Refnum out"=w11:T1)  [unwired: 7 in, 1 out]
    n15 = call "Agilent 34970 Read Continuous.vi"("VISA Resource Name"=w22, "error in (no error)"=w14) -> ("Output Array"=→"Output Data (Numbers Only)":dbl[], "error out"=w12:errorcluster)  [unwired: 10 in, 2 out]
    n16 = call "UTILITY Release Semaphore.vi"("error in (no error)"=w12, "Refnum in"=w11) -> ()  [unwired: 9 in, 1 out]
    "Numeric" <- w19
  }
